vi "EDA(subVI).vi"(1 "Vzorkovací frekvence":dbl, 2 "EDA array":dbl[](array[numeric])) -> (0 "EDA waveform":waveform(dbl))   [LabVIEW 2026]
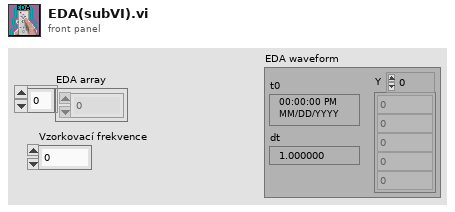
[diagram p1: front panel]
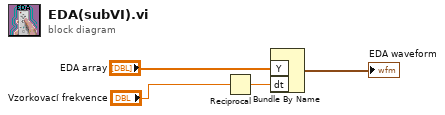
[diagram p0: block diagram]
diagram:
  n1 = Reciprocal(x="Vzorkovací frekvence") -> (1/x=w3:dbl)
  n2 = Bundle By Name("Y"="EDA array", "dt"=w3) -> (→"EDA waveform":waveform(dbl))  [unwired: 1 in]
